vi "Get Hdr Names.vi"() -> ()   [LabVIEW 2010]
panel:
  out "ColHdrString":string[][](array[string])
  in  "Custom Msg":i32(listbox) caption="自定义信息"
  in  "Autotune PID":i32(listbox) caption="PID自动调谐"
  in  "Proc Display":i32(listbox) caption="进度显示"
  in  "Custom Pg":i32(listbox) caption="自定义页"
  in  "System":i32(listbox) caption="系统"
  in  "Main Page":i32(listbox) caption="主界面"
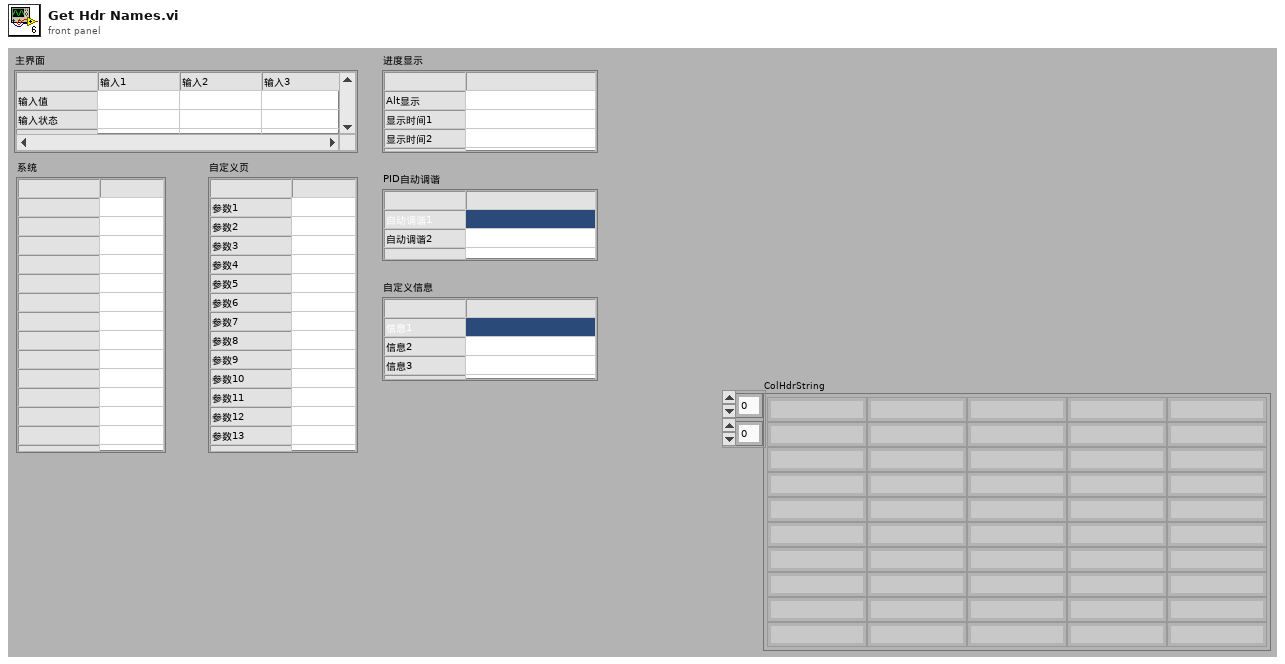
[diagram p1: front panel]
types:
  T1 = enum32{"Invalid", "Standard", "Closed", "Hidden", "Minimized", "Maximized"}
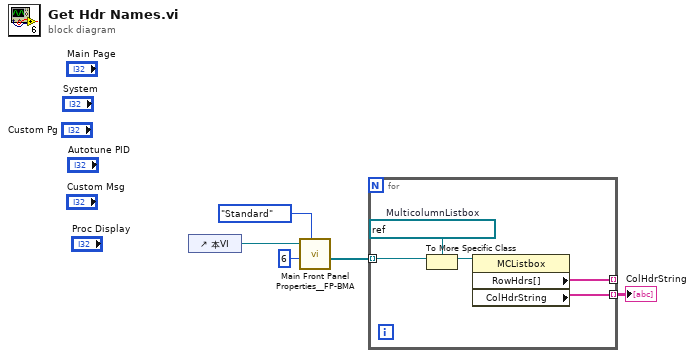
[diagram p0: block diagram]
diagram:
  n1 = control-ref of="本VI"() -> (w5:refnum<vi>)
  n2 = call "Main Front Panel Properties__FP-BMA.vi"("window state"=T1."Standard", "number of Datalist"=6 ("number of DataList"), "VI ref in"=w5) -> ("DataList"=w3:refnum<vi>[])  [unwired: 3 in, 5 out]
  n3 = for {
    tunnel: w3 -> [w10] mode=indexing
    tunnel: [w7] -> _ mode=indexing
    tunnel: [w6] -> w2 mode=indexing
    w8 = refnum<vi> refnum  # MulticolumnListbox
    n4 = To More Specific Class(target class=w8, reference=w10) -> (specific class reference=w9:refnum<vi>)  [unwired: 1 in, 1 out]
    n5 = property class="MCListbox"(reference=w9) -> ("RowHdrs[]"=w7:string[], "ColHdrString"=w6:string[])  [unwired: 1 in, 2 out]
  }
  "ColHdrString" <- w2
